vi "Kinect Extracted Contour Report.vi"(10 "Interval Range":cluster{"Minimum":sgl, "Maximum":sgl}={"Minimum"=0.0, "Maximum"=300.0} {"Maximum" format="%.2f"; "Minimum" format="%.2f"}, 11 "Image":T1) -> (0 "Mean Right Value":sgl format="%.2f", 1 "Mean Left Value":sgl format="%.2f", 2 "Right Histogram":T2(graph), 3 "Left Histogram":T2(graph))   [LabVIEW 2011]
uses:
  <vilib>/vision/Image Controls.llb/IMAQ Image.ctl
  <vilib>/vision/NI_Vision_Development_Module.lvlib
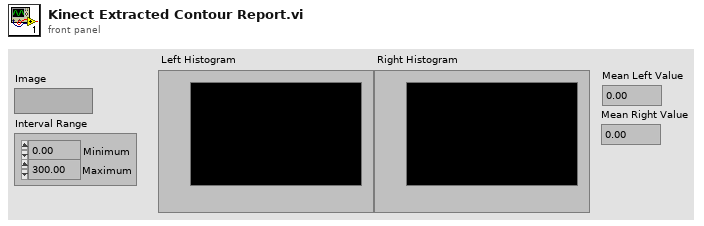
[diagram p1: front panel]
types:
  T1 = typedef "IMAQ Image.ctl" = refnum<image>
  T2 = cluster{"Starting Value":sgl, "Incremental Value":sgl, "Histogram":u32[]}
  T3 = typedef "Image Type" = u32
  T4 = cluster{"Lower value":sgl, "Upper value":sgl, "Replace Value":sgl, "Keep/Replace Value (Replace)":bool}[]
  T5 = typedef "IMAQ Rectangle" = cluster{"Left":i32, "Top":i32, "Right":i32, "Bottom":i32, "Rotation":dbl}
  T6 = typedef "ROI Descriptor" = cluster{"Global Rectangle":i32[], "Contours":cluster{"ID":enum32{"External", "Internal"}, "Type":u32, "Coordinates":i32[]}[]}
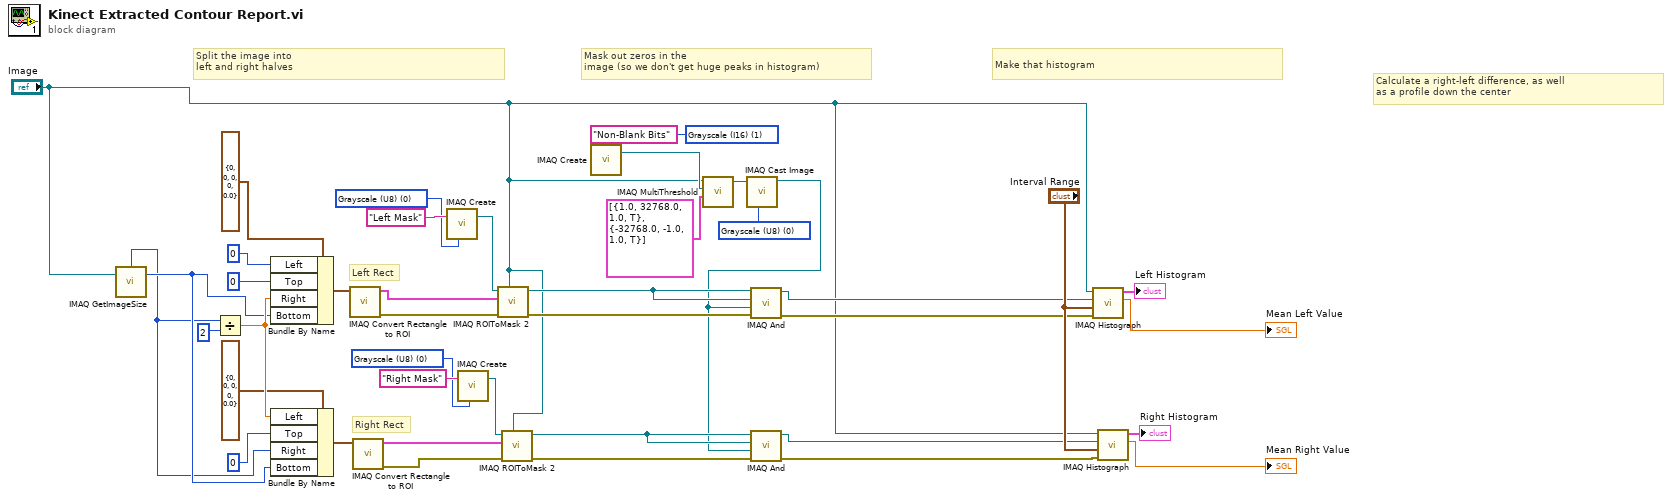
[diagram p0: block diagram]
diagram:
  w3 = T3 0 items=["Grayscale (U8)", "Grayscale (I16)", "Grayscale (SGL)", "Complex (CSG)", "RGB (U32)", "HSL (U32)", "RGB (U64)", "Grayscale (U16)"] ("Image Type")
  w6 = T3 1 items=["Grayscale (U8)", "Grayscale (I16)", "Grayscale (SGL)", "Complex (CSG)", "RGB (U32)", "HSL (U32)", "RGB (U64)", "Grayscale (U16)"] ("Image Type")
  w13 = T3 0 items=["Grayscale (U8)", "Grayscale (I16)", "Grayscale (SGL)", "Complex (CSG)", "RGB (U32)", "HSL (U32)", "RGB (U64)", "Grayscale (U16)"] ("Image Type")
  w14 = T3 0 items=["Grayscale (U8)", "Grayscale (I16)", "Grayscale (SGL)", "Complex (CSG)", "RGB (U32)", "HSL (U32)", "RGB (U64)", "Grayscale (U16)"] ("Image Type")
  # "Calculate a right-left difference, as well\nas a profile down the center"
  # "Make that histogram"
  # "Mask out zeros in the \nimage (so we don't get huge peaks in histogram)"
  # "Split the image into\nleft and right halves"
  # "Right Rect"
  # "Left Rect"
  n1 = call "IMAQ GetImageSize"("Image"="Image") -> ("Y Resolution"=w30:i32, "X Resolution"=w29:i32)  [unwired: 3 in, 1 out]
  n2 = Divide(x=w29, y=2) -> (x/y=w32:dbl)
  n3 = Bundle By Name(cluster=T5 {"Left"=0, "Top"=0, "Right"=0, "Bottom"=0, "Rotation"=0.0} ("Rectangle"), "Left"=0, "Top"=0, "Right"=w32, "Bottom"=w30) -> (w27:T5)
  n4 = Bundle By Name(cluster=T5 {"Left"=0, "Top"=0, "Right"=0, "Bottom"=0, "Rotation"=0.0} ("Rectangle"), "Left"=w32, "Top"=0, "Right"=w29, "Bottom"=w30) -> (w26:T5)
  n5 = call "IMAQ Convert Rectangle to ROI"("Rectangle"=w27) -> ("error out"=w39:errorcluster, "ROI Descriptor"=w40:T6)  [unwired: 8 in]
  n6 = call "IMAQ Convert Rectangle to ROI"("Rectangle"=w26) -> ("error out"=w38:errorcluster, "ROI Descriptor"=w37:T6)  [unwired: 8 in]
  n7 = call "IMAQ Create"("Image Name"="Left Mask", "Image Type"=w14) -> ("New Image"=w23:T1)  [unwired: 3 in, 1 out]
  n8 = call "IMAQ Create"("Image Name"="Right Mask", "Image Type"=w13) -> ("New Image"=w22:T1)  [unwired: 3 in, 1 out]
  n9 = call "IMAQ ROIToMask 2"("Image Model"="Image", "error in (no error)"=w39, "ROI Descriptor"=w40, "Image"=w23) -> ("error out"=w12:errorcluster, "Image Out"=w17:T1)  [unwired: 5 in, 1 out]
  n10 = call "IMAQ ROIToMask 2"("Image Model"="Image", "error in (no error)"=w38, "ROI Descriptor"=w37, "Image"=w22) -> ("error out"=w11:errorcluster, "Image Out"=w18:T1)  [unwired: 5 in, 1 out]
  n11 = call "IMAQ Create"("Image Name"="Non-Blank Bits", "Image Type"=w6) -> ("New Image"=w5:T1)  [unwired: 3 in, 1 out]
  n12 = call "IMAQ MultiThreshold"("Threshold Data"=T4 [{"Lower value"=1.0, "Upper value"=32768.0, "Replace Value"=1.0, "Keep/Replace Value (Replace)"=TRUE}, {"Lower value"=-32768.0, "Upper value"=-1.0, "Replace Value"=1.0, "Keep/Replace Value (Replace)"=TRUE}], "Image Dst"=w5, "Image Src"="Image") -> ("Image Dst Out"=w4:T1)  [unwired: 2 in, 1 out]
  n13 = call "IMAQ Cast Image"("Image Type"=w3, "Image Src"=w4) -> ("Image Dst Out"=w2:T1)  [unwired: 8 in, 1 out]
  n14 = call "IMAQ And"("error in (no error)"=w12, "Image Src B"=w2, "Image Dst"=w17, "Image Src A"=w17) -> ("error out"=w10:errorcluster, "Image Dst Out"=w19:T1)  [unwired: 6 in]
  n15 = call "IMAQ And"("error in (no error)"=w11, "Image Src B"=w2, "Image Dst"=w18, "Image Src A"=w18) -> ("error out"=w9:errorcluster, "Image Dst Out"=w20:T1)  [unwired: 6 in]
  n16 = call "IMAQ Histograph"("error in (no error)"=w10, "Interval Range"="Interval Range", "Image Mask"=w19, "Image"="Image") -> ("Mean Value"=→"Mean Left Value":sgl, "Histogram Graph"=→"Left Histogram":T2)  [unwired: 1 in, 5 out]
  n17 = call "IMAQ Histograph"("error in (no error)"=w9, "Interval Range"="Interval Range", "Image Mask"=w20, "Image"="Image") -> ("Mean Value"=→"Mean Right Value":sgl, "Histogram Graph"=→"Right Histogram":T2)  [unwired: 1 in, 5 out]
